vi "robot2.vi"() -> ()   [LabVIEW 2014]
doc: "Use this template to build a producer/consumer design pattern. Use this template when you need to execute a process, such as data analysis, when a data source, such as a triggered acquisition, produces data at an uneven rate and you need to execute the process when the data becomes available."
uses:
  <vilib>/picture/picture.llb/imagedata.ctl
  <vilib>/Utility/miscctls.llb/LVBoundsTypeDef.ctl
panel:
  in  "Draw Area Size":T1
  out "2D Picture":picture
  out "Distance":i32
  in  "stop":bool
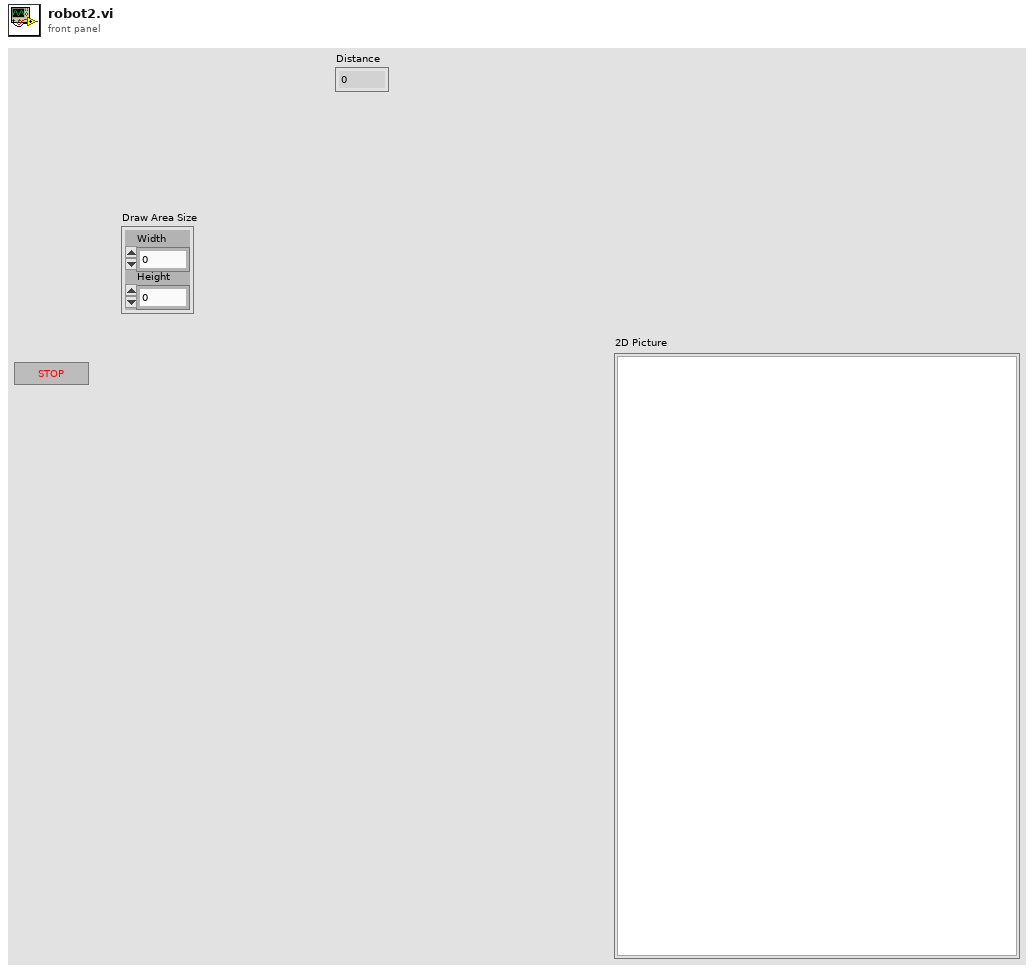
[diagram p1: front panel]
types:
  T1 = typedef "LVBoundsTypeDef.ctl" = cluster{"Width":u32, "Height":u32}
  T2 = cluster{"maximum":dbl, "minimum":dbl, "clip to min":bool, "log?(F)":bool, "grid color":u32, "plot color":u32, "fmt and prec":cluster{"format":enum8{"Decimal", "Scientific", "Engineering", "Binary", "Octal", "Hex"}, "precision":u8}, "visible section":u16}
  T3 = typedef "imagedata.ctl" = cluster{"image type":i32, "image depth":i32, "image":u8[], "mask":u8[], "colors":u32[], "Rectangle":cluster{"left":i16, "top":i16, "right":i16, "bottom":i16}}
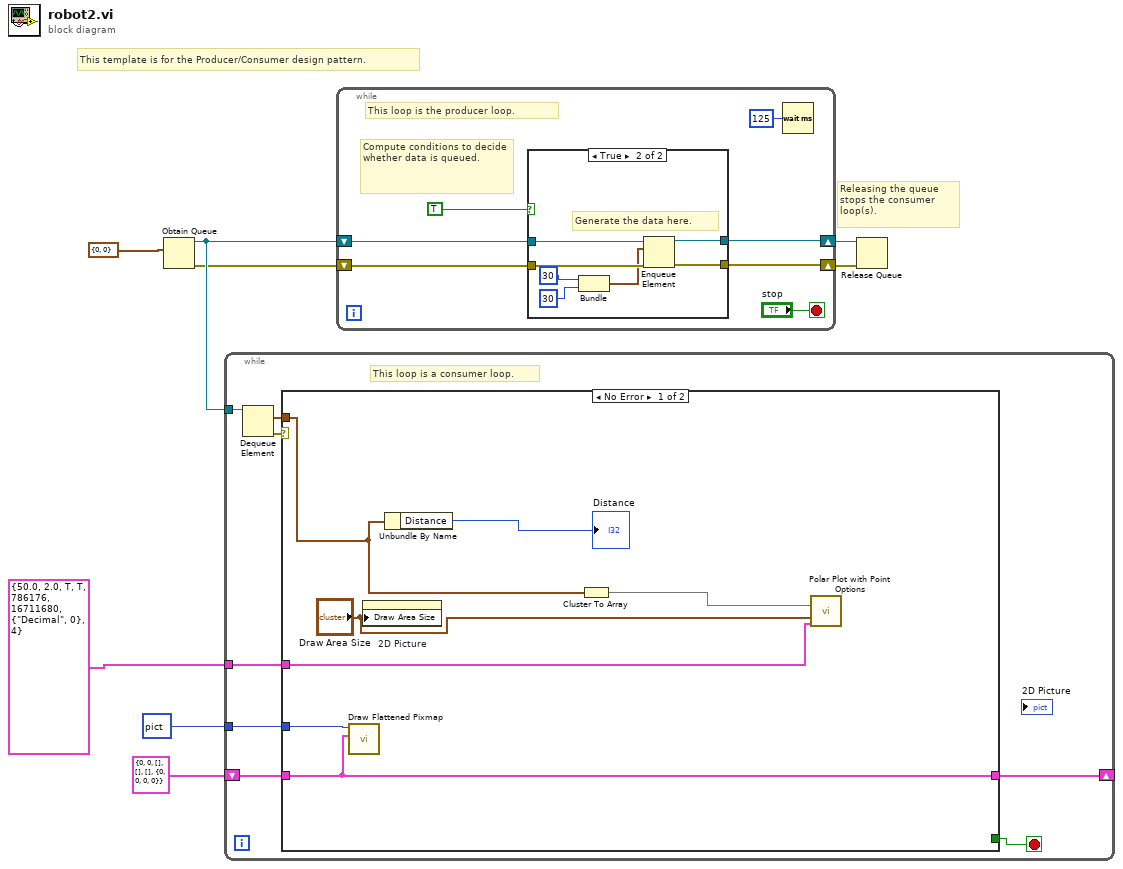
[diagram p0: block diagram]
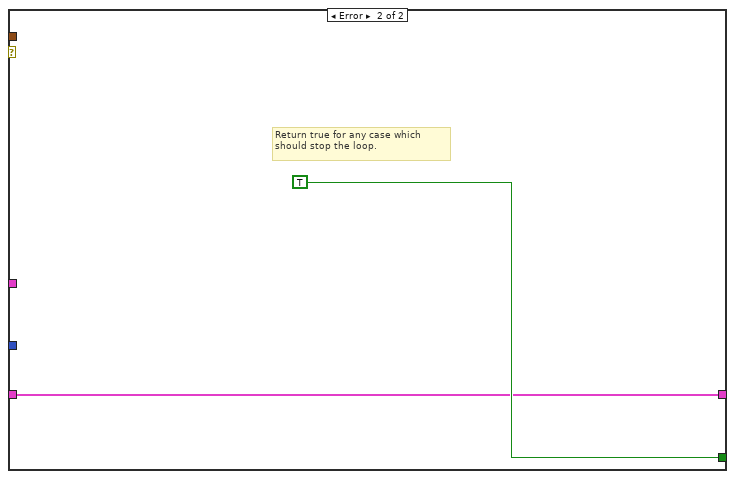
[diagram p2: hidden frame]
diagram:
  # "Releasing the queue stops the consumer loop(s)."
  # "This template is for the Producer/Consumer design pattern."
  n1 = Obtain Queue(element data type=cluster{"Distance":i32, "Angle":i32} {"Distance"=0, "Angle"=0}) -> (queue out=w8:refnum<queue>, error out=w7:errorcluster)  [unwired: 4 in, 1 out]
  n2 = while {
    tunnel: w8 -> [w16]
    tunnel: picture data[5B] ("picture") -> [w12]
    shift-right: [w10] -> _
    shift-left: T3 {"image type"=0, "image depth"=0, "image"=[], "mask"=[], "colors"=[], "Rectangle"={"left"=0, "top"=0, "right"=0, "bottom"=0}} ("image data") -> [w11]
    tunnel: T2 {"maximum"=50.0, "minimum"=2.0, "clip to min"=TRUE, "log?(F)"=TRUE, "grid color"=786176, "plot color"=16711680, "fmt and prec"={"format"=enum."Decimal", "precision"=0}, "visible section"=4} ("polar attributes") -> [w9]
    stop <- w13 stop-if-true
    # "This loop is a consumer loop."
    n3 = Dequeue Element(queue=w16) -> (element=w14:cluster{"Distance":i32, "Angle":i32}, error out=w15:errorcluster)  [unwired: 2 in, 2 out]
    n4 = case shown="No Error" w15 {
      tunnel: w14 -> [w17 _]
      tunnel: [_ TRUE] -> w13
      tunnel: w12 -> [w22 _]
      tunnel: w11 -> [w21 w24]
      tunnel: [w21 w24] -> w10
      tunnel: w9 -> [w20 _]
      frame No Error {
        n5 = call <vilib>:"Draw Flattened Pixmap.vi"("image data"=w21, "picture"=w22) -> ()  [unwired: 7 in, 1 out]
        n6 = property on="2D Picture" class="Pict"("Draw Area Size"="Draw Area Size") -> ()  [unwired: 2 in, 2 out]
        n7 = Unbundle By Name(w17) -> ("Distance"=→"Distance":i32)
        n8 = Cluster To Array(cluster=w17) -> (array=w18:i32[])
        n9 = call <vilib>:"Polar Plot with Point Options.vi"("data array [mag, phase (deg)]"=w18, "dimensions (w,h)"="Draw Area Size", "polar attributes"=w20) -> ()  [unwired: 12 in, 1 out]
      }
      frame Error {
        # "Return true for any case which should stop the loop."
      }
    }
  }
  n10 = while {
    shift-right: [w28] -> w5
    shift-left: w7 -> [w29]
    shift-right: [w30] -> w6
    shift-left: w8 -> [w31]
    stop <- "stop" stop-if-true
    # "Compute conditions to decide whether data is queued."
    # "This loop is the producer loop."
    n11 = case shown="True" TRUE ("Case Constant\n(See Context Help)") {
      tunnel: w31 -> [w34 w41]
      tunnel: [w34 w40] -> w30
      tunnel: w29 -> [w33 w39]
      tunnel: [w33 w38] -> w28
      frame False {
      }
      frame True {
        # "Generate the data here."
        n12 = Bundle(30, 30) -> (w35:cluster{i32, i32})  [unwired: 1 in]
        n13 = Enqueue Element(queue=w41, element=w35, error in (no error)=w39) -> (queue out=w40:refnum<queue>, error out=w38:errorcluster)  [unwired: 1 in, 1 out]
      }
    }
    n14 = Wait (ms)(milliseconds to wait=u32 125) -> ()  [unwired: 1 out]
  }
  n15 = Release Queue(queue=w6, error in (no error)=w5) -> ()  [unwired: 1 in, 3 out]
